vi "Setup UI.vi"(8 "error in (no error)":errorcluster, 10 "Set UI to input? (F)":bool, 11 "Keithley Multimeter in":refnum<class "Keithley Multimeter.lvclass">) -> (0 "error out":errorcluster, 3 "Keithley Multimeter out":refnum<class "Keithley Multimeter.lvclass">)   [LabVIEW 2017, in "Keithley Multimeter.lvclass"]
doc: "Setup UI constructs an object -- populates its member fields -- from a front panel the user can see. The VI should be as simple as possible so that a UI loop can poll it continuously for updates. \n\nThe VI is designed to be used as a subPanel within another VI. Wire true to \"Set UI to input\" only on the first call, just after inserting this VI into a subPanel, to populate its controls with the class's current values.\n\nSetup UI is distinct from the class constructor. Class constructors are not polymorphic, yet configure dialogs need to configure objects without knowing their type -- and polymorphism is the necessary solution. Thus, Setup UI is a polymorphic class constructor. This continously polled \"Setup UI\" concept is a kludge: a better idea would be an XControl, but those require a steeper learning curve."
uses:
  Keithley Multimeter.lvclass
  Keithley Multimeter.lvclass/Keithley Multimeter.ctl
  Utility Classes/Readable/Readable.lvclass
panel:
  out "Tab Control":enum32{"0", "1", "2", "3", "4", "5", "6", "7"}(tab)
  in  "AC Voltage Configuration":T1={"dBm ref impedance (75:1)"=1, "peak window (secs)"=0.1, "detector (rms:0)"=0, "dB reference (volts)"=1.0, "AC voltage (volts:0)"=0, "reference value (volts)"=0.0, "range value (volts)"=750.0} {"range value (volts)" min=0.2 max=750.0 format="%^.2e"; "reference value (volts)" min=-775.0 max=775.0 format="%^.2e"; "AC voltage (volts:0)" items=["volts", "DB", "DBM"]; "dB reference (volts)" min=0.001 max=750.0 format="%.3f"; "detector (rms:0)" items=["RMS", "average", "low frequency RMS", "AC peak voltage", "DC negative peak spike", "DC positive peak spike"]; "peak window (secs)" min=0.1 max=9.9 format="%.2f"; "dBm ref impedance (75:1)" items=["50 ohms", "75 ohms", "93 ohms", "132 ohms", "300 ohms", "600 ohms"]}
  in  "DC Voltage Configuration":T2={"reference value (volts)"=0.0, "range value (volts)"=1000.0} {"range value (volts)" min=0.2 max=1000.0 format="%^.2e"; "reference value (volts)" min=-1100.0 max=1100.0 format="%^.2e"}
  in  "2 Wire Resistance Configuration":T3={"offset compensation"=FALSE, "reference value (ohms)"=0.0, "range value (ohms)"=1000000000.0} {"range value (ohms)" min=20.0 max=1000000000.0 format="%^.2e"; "reference value (ohms)" min=-1000000000.0 max=1000000000.0 format="%^.2e"}
  in  "4 Wire Resistance Configuration":T3={"offset compensation"=FALSE, "reference value (ohms)"=0.0, "range value (ohms)"=200000.0} {"range value (ohms)" min=20.0 max=200000.0 format="%^.2e"; "reference value (ohms)" min=-200000.0 max=200000.0 format="%^.2e"}
  in  "AC Current Configuration":T4={"detector (rms:0)"=0, "reference value (amps)"=0.0, "range value (amps)"=2.0} {"range value (amps)" min=0.0002 max=2.0 format="%^.2e"; "reference value (amps)" min=-2.1 max=2.1 format="%^.2e"; "detector (rms:0)" items=["RMS", "average"]}
  in  "DC Current Configuration":T5={"reference value (amps)"=0.0, "method"=TRUE, "range value (amps)"=2.0} {"range value (amps)" min=0.0002 max=2.0 format="%^.2e"; "reference value (amps)" min=-2.1 max=2.1 format="%^.2e"}
  in  "Frequency Configuration":T6={"source"=FALSE, "resolution (5 digits:1)"=1, "threshold current range (1mA:0)"=0, "reference value (Hz)"=0.0, "threshold current level"=0.0, "threshold voltage range (10V:1)"=1, "threshold voltage level"=0.0} {"threshold voltage level" min=-600.0 max=600.0 step=1.0 format="%^.2e"; "threshold voltage range (10V:1)" items=["1 V", "10 V", "100 V", "1000 V", "TTL"]; "threshold current level" min=-0.6 max=0.6 format="%^.2e"; "reference value (Hz)" min=0.0 max=15000000.0 format="%^.2e"; "threshold current range (1mA:0)" items=["1 mA", "10 mA", "100 mA", "1 A"]; "resolution (5 digits:1)" items=["4 digits", "5 digits"]}
  out "String":string
  in  "function":u16(ring)=1 items=["ac voltage", "dc voltage", "2-wire resistance", "4-wire resistance", "ac current", "dc current", "frequency", "temperature"]
  in  "Configuration Values":T7={"range (auto:0)"=0, "dig. filter count"=10.0, "digital filter (off:0)"=0, "advanced filter (off:0)"=0, "integration time (0:auto)"=0, "integ. value"=0.01667, "resolution (4.5 digits:3)"=3, "noise tolerance (%)"=1.0, "reference (off:0)"=0, "coupling"=TRUE, "function (Vdc:1)"=1} {"function (Vdc:1)" items=["ac voltage", "dc voltage", "2-wire resistance", "4-wire resistance", "ac current", "dc current", "frequency", "temperature"]; "reference (off:0)" items=["off", "set reference value"]; "noise tolerance (%)" min=0.0 max=100.0 step=1.0 format="%^.2e"; "resolution (4.5 digits:3)" items=["auto resolution", "auto resolution once", "3.5 digits", "4.5 digits", "5.5 digits", "6.5 digits", "7.5 digits", "8.5 digits"]; "integ. value" format="%^.2e"; "integration time (0:auto)" items=["automatic", "automatic once", "set to minimum", "set to maximum", "set aperature value", "set NPLC value"]; "advanced filter (off:0)" items=["off", "enabled"]; "digital filter (off:0)" items=["off", "auto filter", "auto filter once", "moving filter", "repeating filter"]; "dig. filter count" min=1.0 max=100.0 step=1.0 format="%^.2e"; "range (auto:0)" items=["autorange", "autorange once", "set min range", "set max range", "set range value"]}
  # "Keithley Setup"
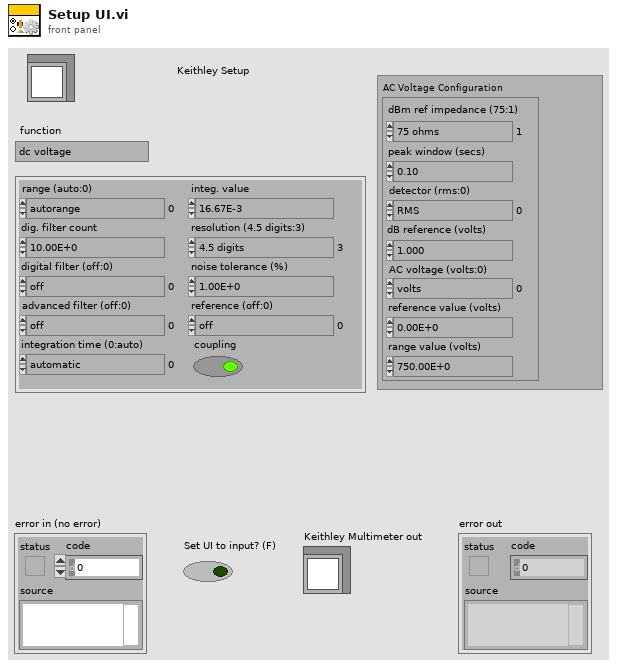
[diagram p1: front panel]
types:
  T1 = cluster{"dBm ref impedance (75:1)":u16, "peak window (secs)":dbl, "detector (rms:0)":u16, "dB reference (volts)":dbl, "AC voltage (volts:0)":u16, "reference value (volts)":dbl, "range value (volts)":dbl}
  T2 = cluster{"reference value (volts)":dbl, "range value (volts)":dbl}
  T3 = cluster{"offset compensation":bool, "reference value (ohms)":dbl, "range value (ohms)":dbl}
  T4 = cluster{"detector (rms:0)":u16, "reference value (amps)":dbl, "range value (amps)":dbl}
  T5 = cluster{"reference value (amps)":dbl, "method":bool, "range value (amps)":dbl}
  T6 = cluster{"source":bool, "resolution (5 digits:1)":u16, "threshold current range (1mA:0)":u16, "reference value (Hz)":dbl, "threshold current level":dbl, "threshold voltage range (10V:1)":u16, "threshold voltage level":dbl}
  T7 = cluster{"range (auto:0)":u16, "dig. filter count":dbl, "digital filter (off:0)":u16, "advanced filter (off:0)":u16, "integration time (0:auto)":u16, "integ. value":dbl, "resolution (4.5 digits:3)":u16, "noise tolerance (%)":dbl, "reference (off:0)":u16, "coupling":bool, "function (Vdc:1)":u16}
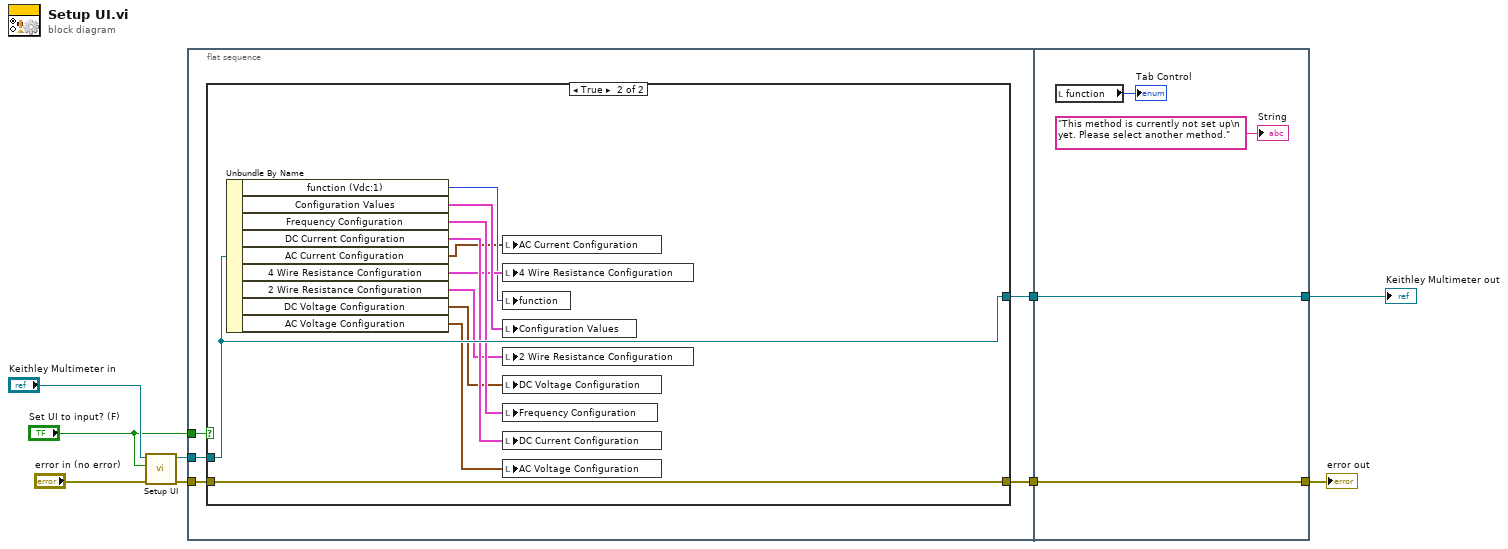
[diagram p0: block diagram]
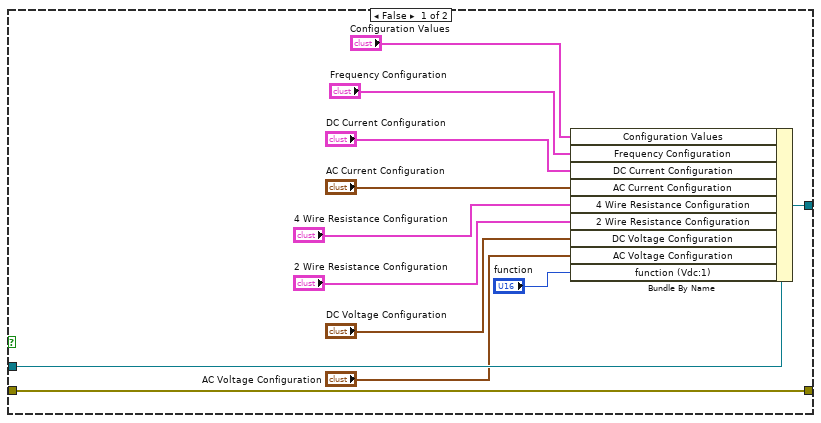
[diagram p2: hidden frame]
diagram:
  n1 = call-parent "Setup UI.vi"("error in (no error)"="error in (no error)", "Set UI to input? (F)"="Set UI to input? (F)", "Instrument in"="Keithley Multimeter in") -> ("error out"=w5:errorcluster, "Instrument out"=w4:refnum<class "Keithley Multimeter.lvclass">)  [unwired: 7 in]
  n2 = flat-sequence {
    tunnel: [w14] -> w7
    tunnel: [w13] -> w6
    tunnel: w5 -> [w12]
    tunnel: w4 -> [w11]
    tunnel: "Set UI to input? (F)" -> [w10]
    tunnel: [w40] -> w2
    tunnel: [w41] -> w3
    tunnel: w7 -> [w41]
    tunnel: w6 -> [w40]
    frame #0 {
      n3 = case shown="True" w10 {
        tunnel: w11 -> [w25 w37]
        tunnel: [w26 w37] -> w14
        tunnel: w12 -> [w15 w36]
        tunnel: [w15 w36] -> w13
        frame False {
          n4 = Bundle By Name(cluster=w25, "Configuration Values"="Configuration Values", "Frequency Configuration"="Frequency Configuration", "DC Current Configuration"="DC Current Configuration", "AC Current Configuration"="AC Current Configuration", "4 Wire Resistance Configuration"="4 Wire Resistance Configuration", "2 Wire Resistance Configuration"="2 Wire Resistance Configuration", "DC Voltage Configuration"="DC Voltage Configuration", "AC Voltage Configuration"="AC Voltage Configuration", "function (Vdc:1)"="function") -> (w26:refnum<class "Keithley Multimeter.lvclass">)
        }
        frame True {
          n5 = Unbundle By Name(w37) -> ("function (Vdc:1)"=w28:u16, "Configuration Values"=w35:T7, "Frequency Configuration"=w34:T6, "DC Current Configuration"=w33:T5, "AC Current Configuration"=w27:T4, "4 Wire Resistance Configuration"=w32:T3, "2 Wire Resistance Configuration"=w31:T3, "DC Voltage Configuration"=w30:T2, "AC Voltage Configuration"=w29:T1)
          n6 = local write "AC Current Configuration"(w27) -> ()
          n7 = local write "4 Wire Resistance Configuration"(w32) -> ()
          n8 = local write "function"(w28) -> ()
          n9 = local write "Configuration Values"(w35) -> ()
          n10 = local write "2 Wire Resistance Configuration"(w31) -> ()
          n11 = local write "DC Voltage Configuration"(w30) -> ()
          n12 = local write "Frequency Configuration"(w34) -> ()
          n13 = local write "DC Current Configuration"(w33) -> ()
          n14 = local write "AC Voltage Configuration"(w29) -> ()
        }
      }
    }
    frame #1 {
      n15 = local read "function"() -> (→"Tab Control":u16)
      "String" <- "This method is currently not set up\n yet. Please select another method." ("String")
    }
  }
  "error out" <- w2
  "Keithley Multimeter out" <- w3
